vi "Create Result Page.vi"(8 "error in (no error)":errorcluster, 9 "Test Results":T1, 10 "Test Info":T3, 11 "Report In":refnum<class "NI_report.lvclass">) -> (0 "error out":errorcluster, 1 "Test Results Out":T1, 2 "Test info Out":T3, 3 "Report Out":refnum<class "NI_report.lvclass">)   [LabVIEW 2014]
uses:
  Tests/Controls/Test Results.ctl
  Tests/Controls/Step Result.ctl
  <vilib>/Utility/NIReport.llb/NI_report.lvclass
  <vilib>/addons/_office/excel.llb/Excel Easy Table (str).vi
  <vilib>/addons/_office/NI_ReportGenerationToolkit.lvlib
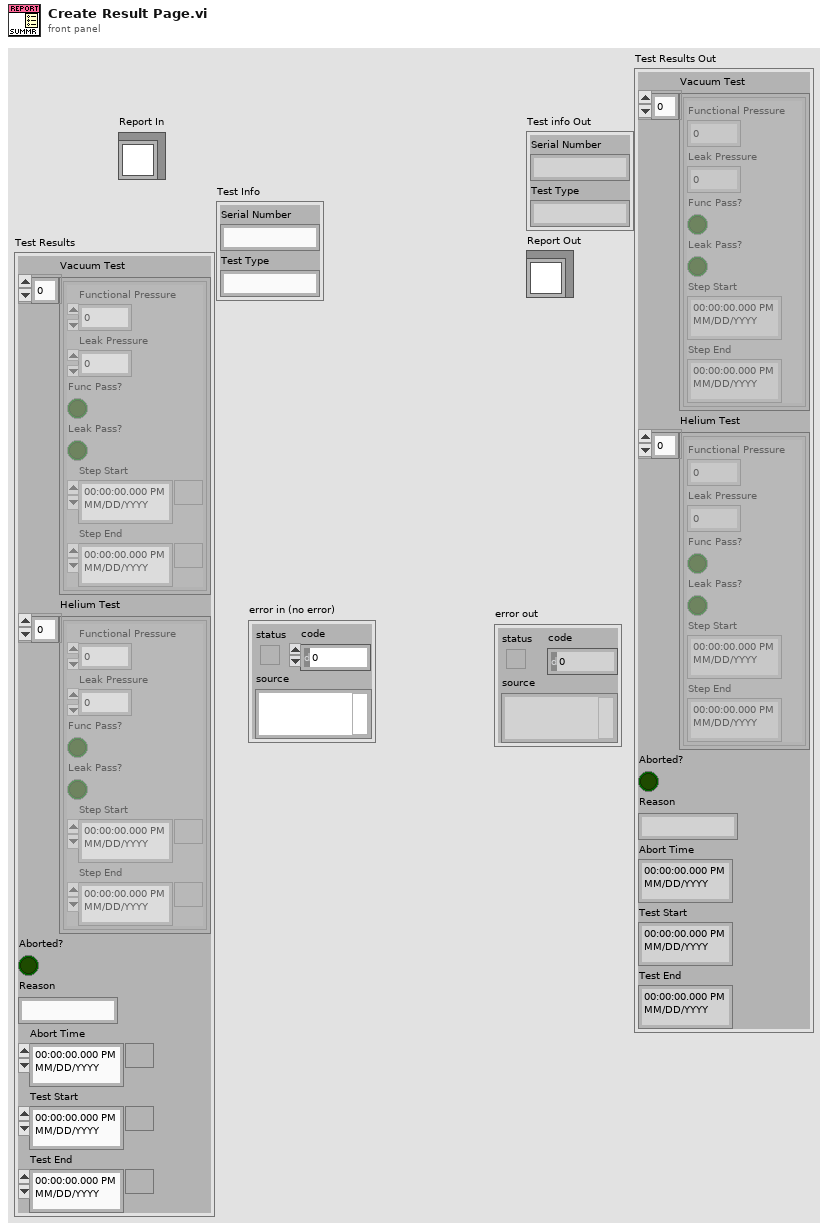
[diagram p1: front panel]
types:
  T1 = typedef "Test Results.ctl" = cluster{"Vacuum Test":T2[], "Helium Test":T2[], "Aborted?":bool, "Reason":string, "Abort Time":timestamp, "Test Start":timestamp, "Test End":timestamp}
  T2 = typedef "Step Result.ctl" = cluster{"Functional Pressure":dbl, "Leak Pressure":dbl, "Func Pass?":bool, "Leak Pass?":bool, "Step Start":timestamp, "Step End":timestamp}
  T3 = cluster{"Serial Number":string, "Test Type":string}
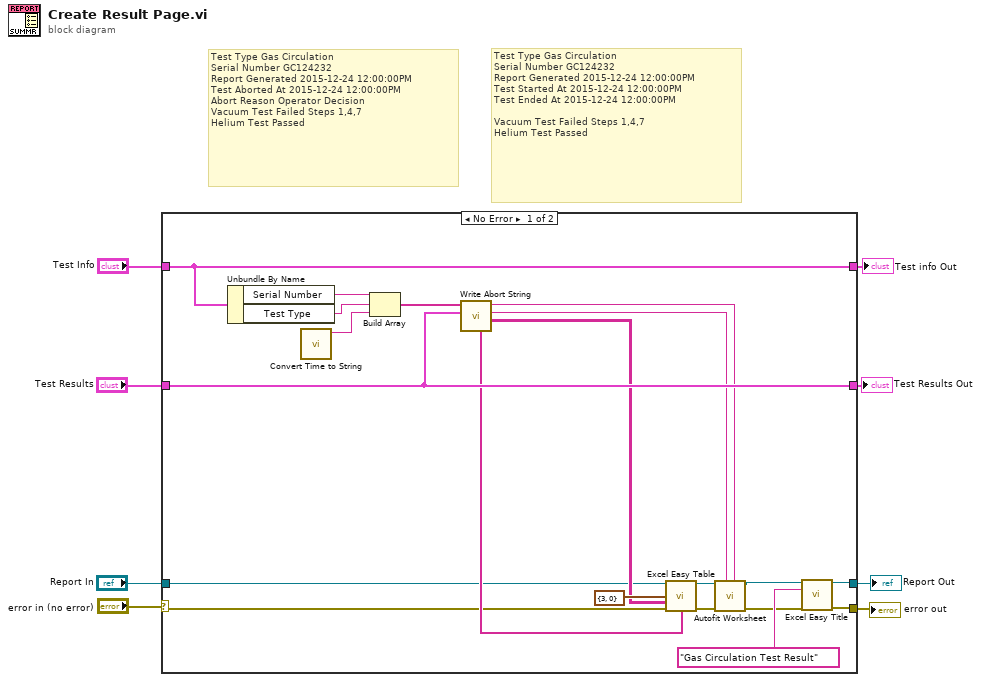
[diagram p0: block diagram]
diagram:
  # "Test Type\tGas Circulation \nSerial Number\tGC124232\nReport Generated\t2015-12-24 12:00:00PM\nTest Started At\t2015-12-24 12:00:00PM\nTest Ended At\t2015-12-24 12:00:00PM\n\nVacuum Test\tFailed Steps 1,4,7\nHelium Test\tPassed"
  # "Test Type\tGas Circulation \nSerial Number\tGC124232\nReport Generated\t2015-12-24 12:00:00PM\nTest Aborted At\t2015-12-24 12:00:00PM\nAbort Reason\tOperator Decision\nVacuum Test\tFailed Steps 1,4,7\nHelium Test\tPassed"
  n1 = case shown="No Error" "error in (no error)" {
    selector: "error in (no error)" -> [w14 w32]
    tunnel: [w9 w32] -> w8
    tunnel: "Test Results" -> [w24 w30]
    tunnel: "Report In" -> [w15 w29]
    tunnel: [w28 w31] -> w3
    tunnel: "Test Info" -> [w28 w31]
    tunnel: [w24 w30] -> w2
    tunnel: [w11 w29] -> w1
    frame No Error {
      n2 = Unbundle By Name(w28) -> ("Serial Number"=w27:string, "Test Type"=w26:string)
      n3 = call "Convert Time to String.vi"() -> ("date/time string"=w25:string)  [unwired: 11 in]
      n4 = Build Array(w27, w26, w25) -> (w23:string[])
      n5 = call "Write Abort String.vi"("Test Results"=w24, "Summary In"=w23) -> ("Summary Out"=w18:string[][], "End Cell"=w16:string, "Start Cell"=w17:string, "Row Headers"=w19:string[])  [unwired: 6 in]
      n6 = call-poly <vilib>:"Excel Easy Table.vi"("report in"=w15, "start (0, 0)"=cluster{"row":i32, "column":i32} {"row"=3, "column"=0}, "text data"=w18, "error in (no error)"=w14, "row headers"=w19) -> ("report out"=w20:refnum<class "NI_report.lvclass">, "error out"=w21:errorcluster)  [unwired: 6 in, 3 out]
      n7 = call "Autofit Worksheet.vi"("Start Cell"=w17, "End Cell"=w16, "error in (no error)"=w21, "Report In"=w20) -> ("error out"=w10:errorcluster, "Report Out"=w12:refnum<class "NI_report.lvclass">)  [unwired: 6 in]
      n8 = call <vilib>:"Excel Easy Title.vi"("report in"=w12, "title"="Gas Circulation Test Result", "error in (no error)"=w10) -> ("report out"=w11:refnum<class "NI_report.lvclass">, "error out"=w9:errorcluster)  [unwired: 10 in, 1 out]
    }
    frame Error {
    }
  }
  "error out" <- w8
  "Test info Out" <- w3
  "Test Results Out" <- w2
  "Report Out" <- w1
